vi "LeCroy.Read.vi"   [LabVIEW 2018]
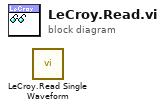
[diagram p0: block diagram]
diagram:
  n1 = call "LeCroy.Read Single Waveform.vi"() -> ()  [unwired: 9 in, 3 out]
